vi "RobotMain.vi"() -> ()   [LabVIEW 2014]
uses:
  <vilib>/myRIO/Instrument Drivers/Utilities/Utilities.lvlib
  <vilib>/ErrorRing/Error Ring.xnode
  DataHighway.ctl
  P:/+Courses/ENGR_3390_Robotics_I/ENGR3390_Fall_2015/For Justin/Project 5 Act Lab Code 2015/DataHighway.ctl
  P:/+Courses/ENGR_3390_Robotics_I/ENGR3390_Fall_2015/For Justin/Project 5 Act Lab Code 2015/Command.ctl
  Command.ctl
panel:
  out "DataHWay":T1
  out "ComHWayFromOCU":T2 {"Speed" scale=-2.0..10.0; "Rudder" scale=-10.0..10.0}
  in  "stop robot control":bool
  out "error out":errorcluster
  # "Robot will run headless\nwithout a control panel\nso keep this control panel\nas simple as possible while\nstill allowing debugging."
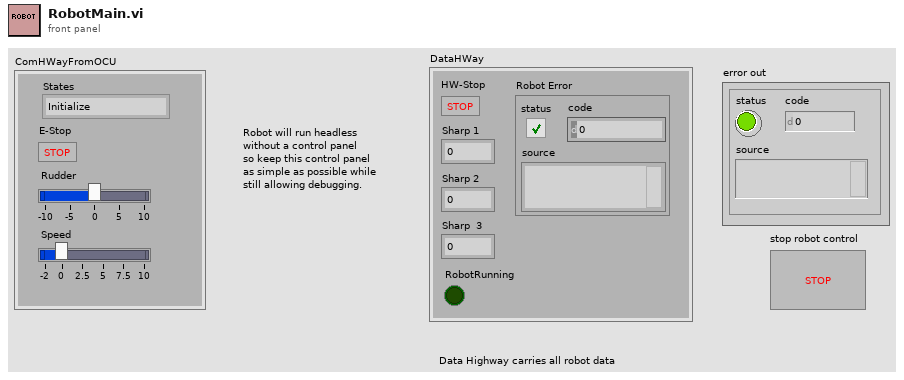
[diagram p1: front panel]
types:
  T1 = typedef "DataHighway.ctl" = cluster{"HW-Stop":bool, "Sharp 1":dbl, "Sharp 2":dbl, "Sharp  3":dbl, "RobotRunning":bool, "Robot Error":errorcluster}
  T2 = typedef "Command.ctl" = cluster{"States":enum16{"Initialize", "Wait for Event", "Debug Robot", "Run Robot", "Exit"}, "E-Stop":bool, "Rudder":dbl, "Speed":dbl}
  T3 = enum16{"Initialize", "Wait for Event", "Debug Robot", "Run Robot", "Exit"}
  T4 = cluster{"Port":dbl, "Center":dbl, "Starboard":dbl}
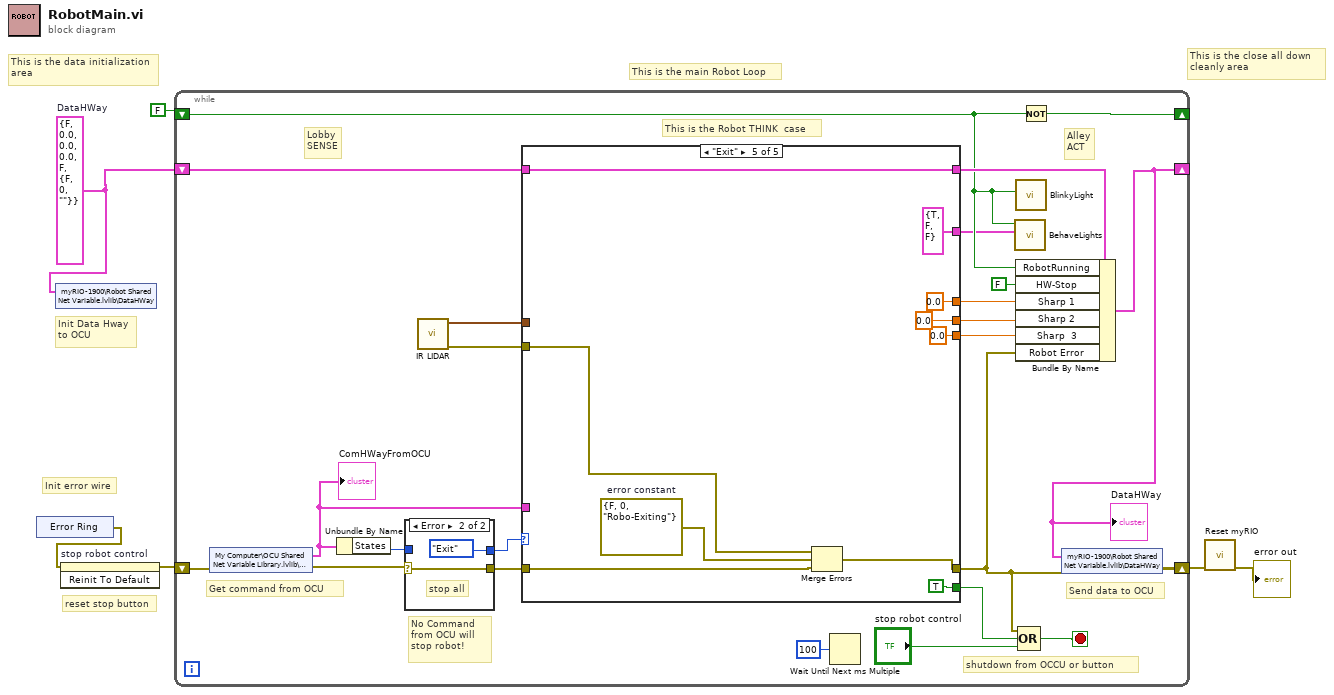
[diagram p0: block diagram]
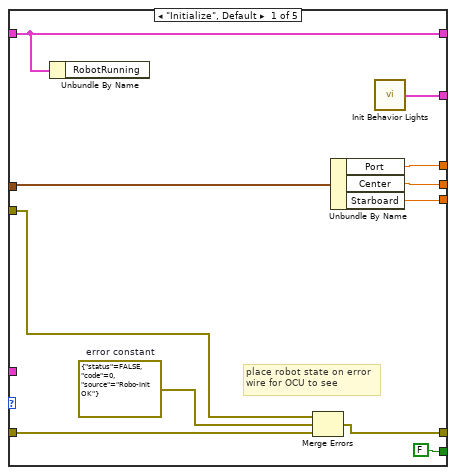
[diagram p3: hidden frame]
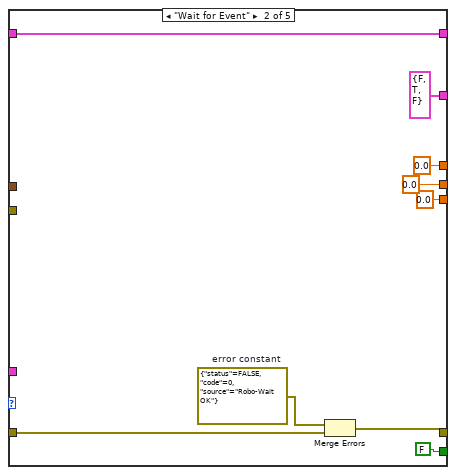
[diagram p4: hidden frame]
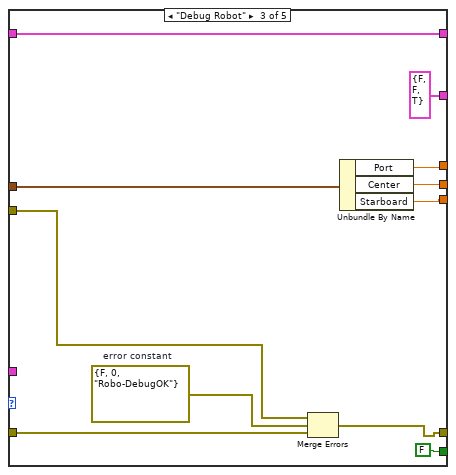
[diagram p5: hidden frame]
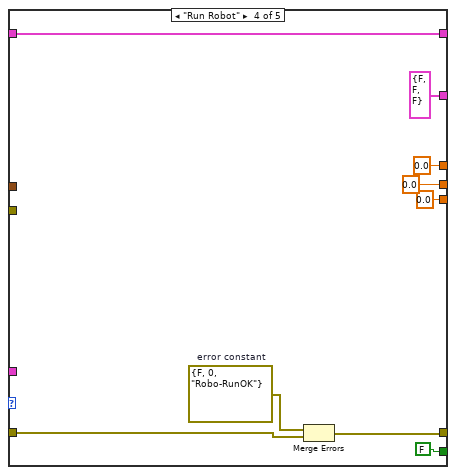
[diagram p6: hidden frame]
diagram:
  w3 = T1 {"HW-Stop"=FALSE, "Sharp 1"=0.0, "Sharp 2"=0.0, "Sharp  3"=0.0, "RobotRunning"=FALSE, "Robot Error"={"status"=FALSE, "code"=0, "source"=""}}  # DataHWay
  # "reset stop button"
  # "Init error wire"
  # "Init Data Hway\nto OCU"
  # "This is the close all down \ncleanly area"
  # "This is the data initialization\narea"
  # "This is the main Robot Loop"
  n1 = xnode "Error Ring"() -> ("error out"=w2:errorcluster)
  n2 = shared-variable "myRIO-1900\\Robot Shared Net Variable.lvlib\\DataHWay"(w3) -> ()  [unwired: 1 in, 1 out]
  n3 = invoke on="stop robot control" class="Bool" method="Reinit To Default"(error in=w2) -> (error out=w1:errorcluster)  [unwired: 2 in, 2 out]
  n4 = while {
    shift-right: [w21] -> w5
    shift-left: w1 -> [w18]
    shift-right: [w16] -> _
    shift-left: w3 -> [w25]
    shift-right: [w20] -> _
    shift-left: FALSE -> [w13]
    stop <- w28 stop-if-true
    # "No Command \nfrom OCU will\nstop robot!"
    # "Get command from OCU"
    # "Send data to OCU"
    # "shutdown from OCCU or button"
    # "Alley\nACT"
    # "This is the Robot THINK  case"
    # "Lobby\nSENSE"
    n5 = shared-variable "My Computer\\OCU Shared Net Variable Library.lvlib\\ComHWay"(error in=w18) -> (w22:T2, error out=w17:errorcluster)
    "ComHWayFromOCU" <- w22
    n6 = Unbundle By Name(w22) -> ("States"=w23:T3)
    n7 = case shown="Error" w17 {
      selector: w17 -> [w32 w34]
      tunnel: [w32 w34] -> w29
      tunnel: [w31 T3."Exit" ("States")] -> w30
      tunnel: w23 -> [w31 _]
      frame No Error {
      }
      frame Error {
        # "stop all"
      }
    }
    n8 = call "IR LIDAR.vi"() -> ("error out"=w10:errorcluster, "Range"=w11:T4)  [unwired: 10 in]
    n9 = case shown="\"Exit\"" w30 {
      tunnel: w29 -> [w44 w52 w63 w72 w82]
      tunnel: [w43 w51 w62 w71 w81] -> w15
      tunnel: [FALSE FALSE FALSE FALSE TRUE] -> w27
      tunnel: w25 -> [w41 w53 w65 w74 w83]
      tunnel: [w41 w53 w65 w74 w83] -> w19
      tunnel: w22 -> [_ _ _ _ _]
      tunnel: [w40 cluster{"Red":bool, "Blue":bool, "Green":bool} {"Red"=FALSE, "Blue"=TRUE, "Green"=FALSE} ("Lights Out") cluster{"Red":bool, "Blue":bool, "Green":bool} {"Red"=FALSE, "Blue"=FALSE, "Green"=TRUE} ("Lights Out") cluster{"Red":bool, "Blue":bool, "Green":bool} {"Red"=FALSE, "Blue"=FALSE, "Green"=FALSE} ("Lights Out") cluster{"Red":bool, "Blue":bool, "Green":bool} {"Red"=TRUE, "Blue"=FALSE, "Green"=FALSE} ("Lights Out")] -> w12
      tunnel: w11 -> [w38 _ w59 _ _]
      tunnel: w10 -> [w39 _ w55 _ w75]
      tunnel: [w37 0.0 ("Port") w58 0.0 ("Port") 0.0 ("Port")] -> w9
      tunnel: [w36 0.0 ("Center") w57 0.0 ("Center") 0.0 ("Center")] -> w8
      tunnel: [w35 0.0 ("Starboard") w56 0.0 ("Starboard") 0.0 ("Starboard")] -> w7
      frame "Initialize", Default {
        w42 = errorcluster {"status"=FALSE, "code"=0, "source"="Robo-Init OK"}  # error constant
        # "place robot state on error\nwire for OCU to see"
        n10 = Unbundle By Name "Unbundle By Name"(w41) -> ()  [unwired: 1 out]
        n11 = Merge Errors "Merge Errors"(w39, w42, w44) -> (w43:errorcluster)
        n12 = Unbundle By Name(w38) -> ("Port"=w37:dbl, "Center"=w36:dbl, "Starboard"=w35:dbl)
        n13 = call "Init Behavior Lights.vi"() -> ("Lights Out"=w40:cluster{"Red":bool, "Blue":bool, "Green":bool})  [unwired: 11 in]
      }
      frame "Wait for Event" {
        w50 = errorcluster {"status"=FALSE, "code"=0, "source"="Robo-Wait OK"}  # error constant
        n14 = Merge Errors "Merge Errors"(w50, w52) -> (w51:errorcluster)
      }
      frame "Debug Robot" {
        w61 = errorcluster {"status"=FALSE, "code"=0, "source"="Robo-DebugOK"}  # error constant
        n15 = Merge Errors "Merge Errors"(w55, w61, w63) -> (w62:errorcluster)
        n16 = Unbundle By Name(w59) -> ("Port"=w58:dbl, "Center"=w57:dbl, "Starboard"=w56:dbl)
      }
      frame "Run Robot" {
        w70 = errorcluster {"status"=FALSE, "code"=0, "source"="Robo-RunOK"}  # error constant
        n17 = Merge Errors "Merge Errors"(w70, w72) -> (w71:errorcluster)
      }
      frame "Exit" {
        w80 = errorcluster {"status"=FALSE, "code"=0, "source"="Robo-Exiting"}  # error constant
        n18 = Merge Errors "Merge Errors"(w75, w80, w82) -> (w81:errorcluster)
      }
    }
    n19 = Wait Until Next ms Multiple(millisecond multiple=u32 100) -> ()  [unwired: 1 out]
    n20 = call "BehaveLights.vi"("BehLightIn"=w12, "Blink"=w13) -> ()  [unwired: 9 in, 1 out]
    n21 = call "BlinkyLight.vi"("Light In"=w13) -> ()  [unwired: 11 in]
    n22 = Bundle By Name(cluster=w19, "RobotRunning"=w13, "HW-Stop"=FALSE, "Sharp 1"=w9, "Sharp 2"=w8, "Sharp  3"=w7, "Robot Error"=w15) -> (w16:T1)
    "DataHWay" <- w16
    n23 = Compound Arithmetic op=OR(w15, w27, "stop robot control") -> (w28:bool)
    n24 = Not(x=w13) -> (.not. x?=w20:bool)
    n25 = shared-variable "myRIO-1900\\Robot Shared Net Variable.lvlib\\DataHWay"(w16, error in=w15) -> (error out=w21:errorcluster)
  }
  n26 = call <vilib>:"Reset myRIO.vi"("error in (no error)"=w5) -> ("error out"=→"error out":errorcluster)  [unwired: 10 in]
